vi "Fit.vi"(8 "error in (no error)":errorcluster caption="entrée d'erreur (pas d'erreur)", 9 "y":string[][](array[string]), 10 "X":string[][](array[string]), 11 "OneHotEncoder.lvclass":refnum<class "OneHotEncoder.lvclass">) -> (0 "error out":errorcluster caption="sortie d'erreur", 2 "String Data":string, 3 "OneHotEncoder.lvclass":refnum<class "OneHotEncoder.lvclass">)   [LabVIEW 2020, in "OneHotEncoder.lvclass"]
doc: "Fit OneHotEncoder to X.\n\nReturns :\n\n- String : OK"
uses:
  OneHotEncoder.lvclass
  OneHotEncoder.lvclass/OneHotEncoder.ctl
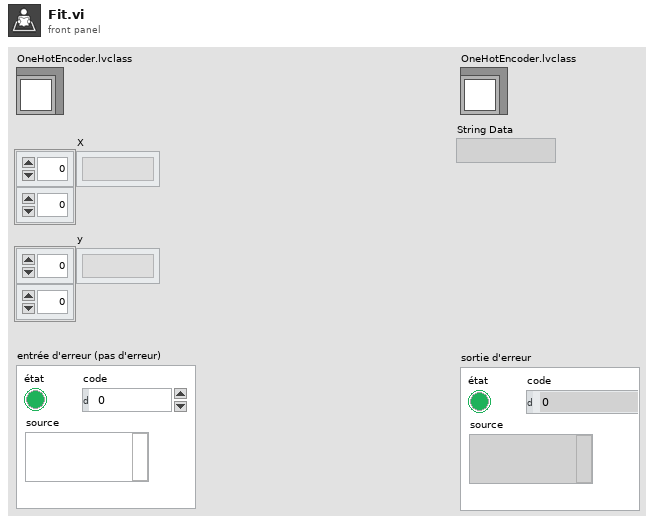
[diagram p1: front panel]
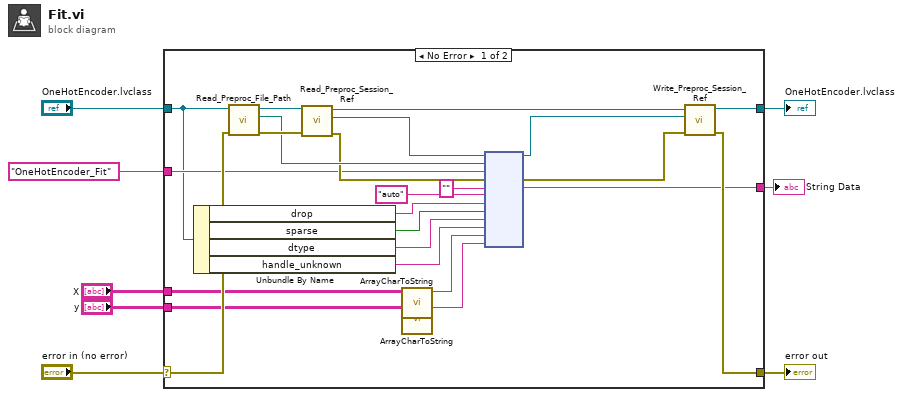
[diagram p0: block diagram]
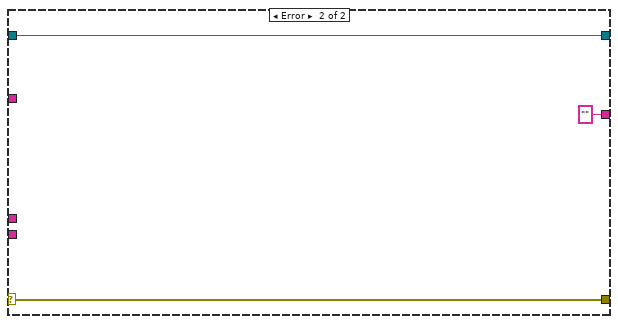
[diagram p2: hidden frame]
diagram:
  n1 = case shown="No Error" "error in (no error)" {
    selector: "error in (no error)" -> [w20 w35]
    tunnel: [w21 w35] -> w7
    tunnel: [w22 w34] -> w5
    tunnel: "OneHotEncoder.lvclass" -> [w17 w34]
    tunnel: "OneHotEncoder_Fit" ("Fonction") -> [w19 _]
    tunnel: [w18 ""] -> w3
    tunnel: "X" -> [w12 _]
    tunnel: "y" -> [w10 _]
    frame No Error {
      n2 = Unbundle By Name(w17) -> ("drop"=w23:string, "sparse"=w15:bool, "dtype"=w14:string, "handle_unknown"=w13:string)
      n3 = call-dynamic "Read_Preproc_File_Path.vi"("error in (no error)"=w20, "Python in"=w17) -> ("error out"=w31:errorcluster, "File_Path"=w28:path, "Python out"=w32:refnum<class "OneHotEncoder.lvclass">)  [unwired: 7 in]
      n4 = call-dynamic "Read_Preproc_Session_Ref.vi"("error in (no error)"=w31, "Python in"=w32) -> ("error out"=w27:errorcluster, "Session_ref"=w29:refnum<k35>, "Python out"=w30:refnum<class "OneHotEncoder.lvclass">)  [unwired: 7 in]
      n5 = call "ArrayCharToString.vi"("TAB"=w12) -> ("Instruction"=w11:string)  [unwired: 10 in]
      n6 = call "ArrayCharToString.vi"("TAB"=w10) -> ("Instruction"=w9:string)  [unwired: 10 in]
      n7 = node(w29, w28, w19, w27, "", "auto", w23, w15, w14, w13, w11, w9) -> (w25:refnum<k35>, w26:errorcluster, w18:string)  [unwired: 7 in, 2 out]
      n8 = call-dynamic "Write_Preproc_Session_Ref.vi"("error in (no error)"=w26, "Session_ref"=w25, "Python in"=w30) -> ("error out"=w21:errorcluster, "Python out"=w22:refnum<class "OneHotEncoder.lvclass">)  [unwired: 7 in]
    }
    frame Error {
    }
  }
  "error out" <- w7
  "OneHotEncoder.lvclass" <- w5
  "String Data" <- w3
